vi "AOI - PCB.vi"() -> ()   [LabVIEW 2017]
doc: "Printed Circuit Board Inspection\nDetermine whether PCB components are present and in the correct location using pattern matching. Match areas of inspection to a template of valid components. Use shift-invariant matching to inspect an oriented component (diode). Use rotation-invariant matching to inspect an unoriented component (resistor)."
panel:
  out "Image":T1(plugin-control)
  out "Not found 1":bool
  out "Not found 2":bool
  out "Number of Matches 2":i32
  out "Number of Matches1":i32
  in  "Template File path 1":path=path "c:/vision/AOI/Template Diode.png"
  in  "Template File path 2":path=path "c:/vision/AOI/Template Resistor.png"
  in  "Image File path":path=path "c:/vision/AOI/SMD Diodes 01.jpg"
  out "Image Log path":path=path "c:/vision/Result.jpg"
  out "error out":errorcluster
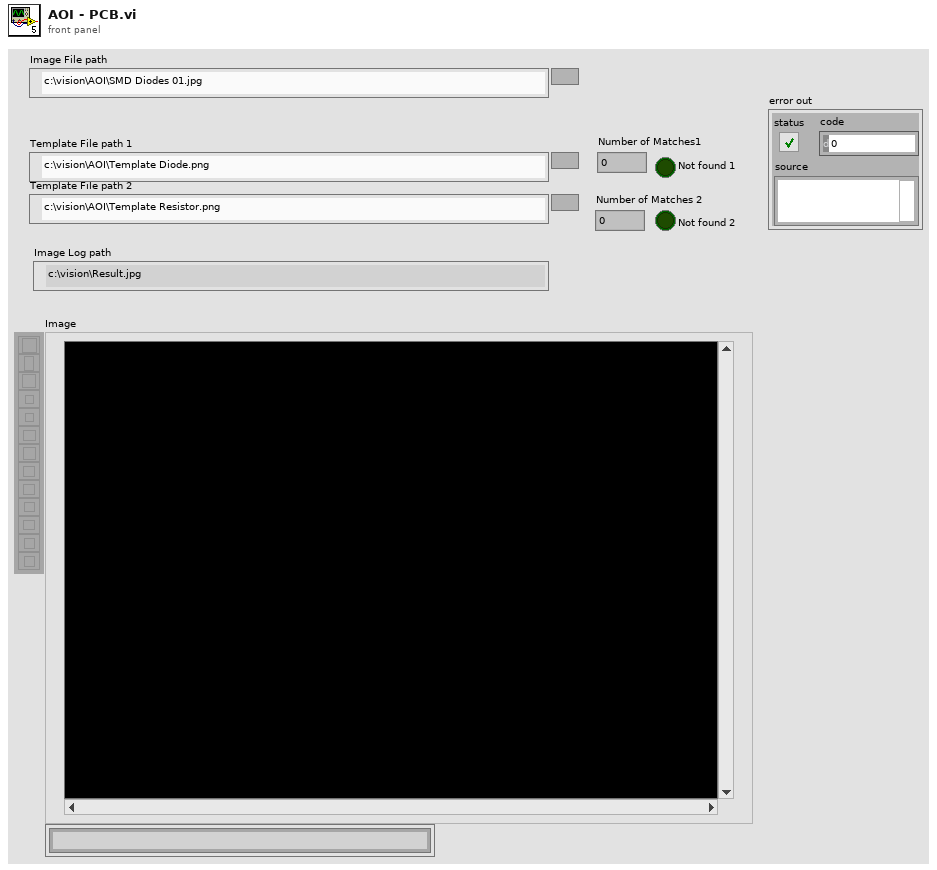
[diagram p1: front panel]
types:
  T1 = typedef "IMAQ Image.ctl" = refnum<image>
  T2 = cluster{"Global Rectangle":i32[], "Contours":cluster{"ID":enum32{"External", "Internal"}, "Type":u32, "Coordinates":i32[]}[]}
  T3 = typedef "Image Type" = u32
  T4 = cluster{"Position":cluster{"x":sgl, "y":sgl}, "Angle":sgl, "Scale":sgl, "Score":sgl, "Bounding Box":cluster{"x":sgl, "y":sgl}[]}[]
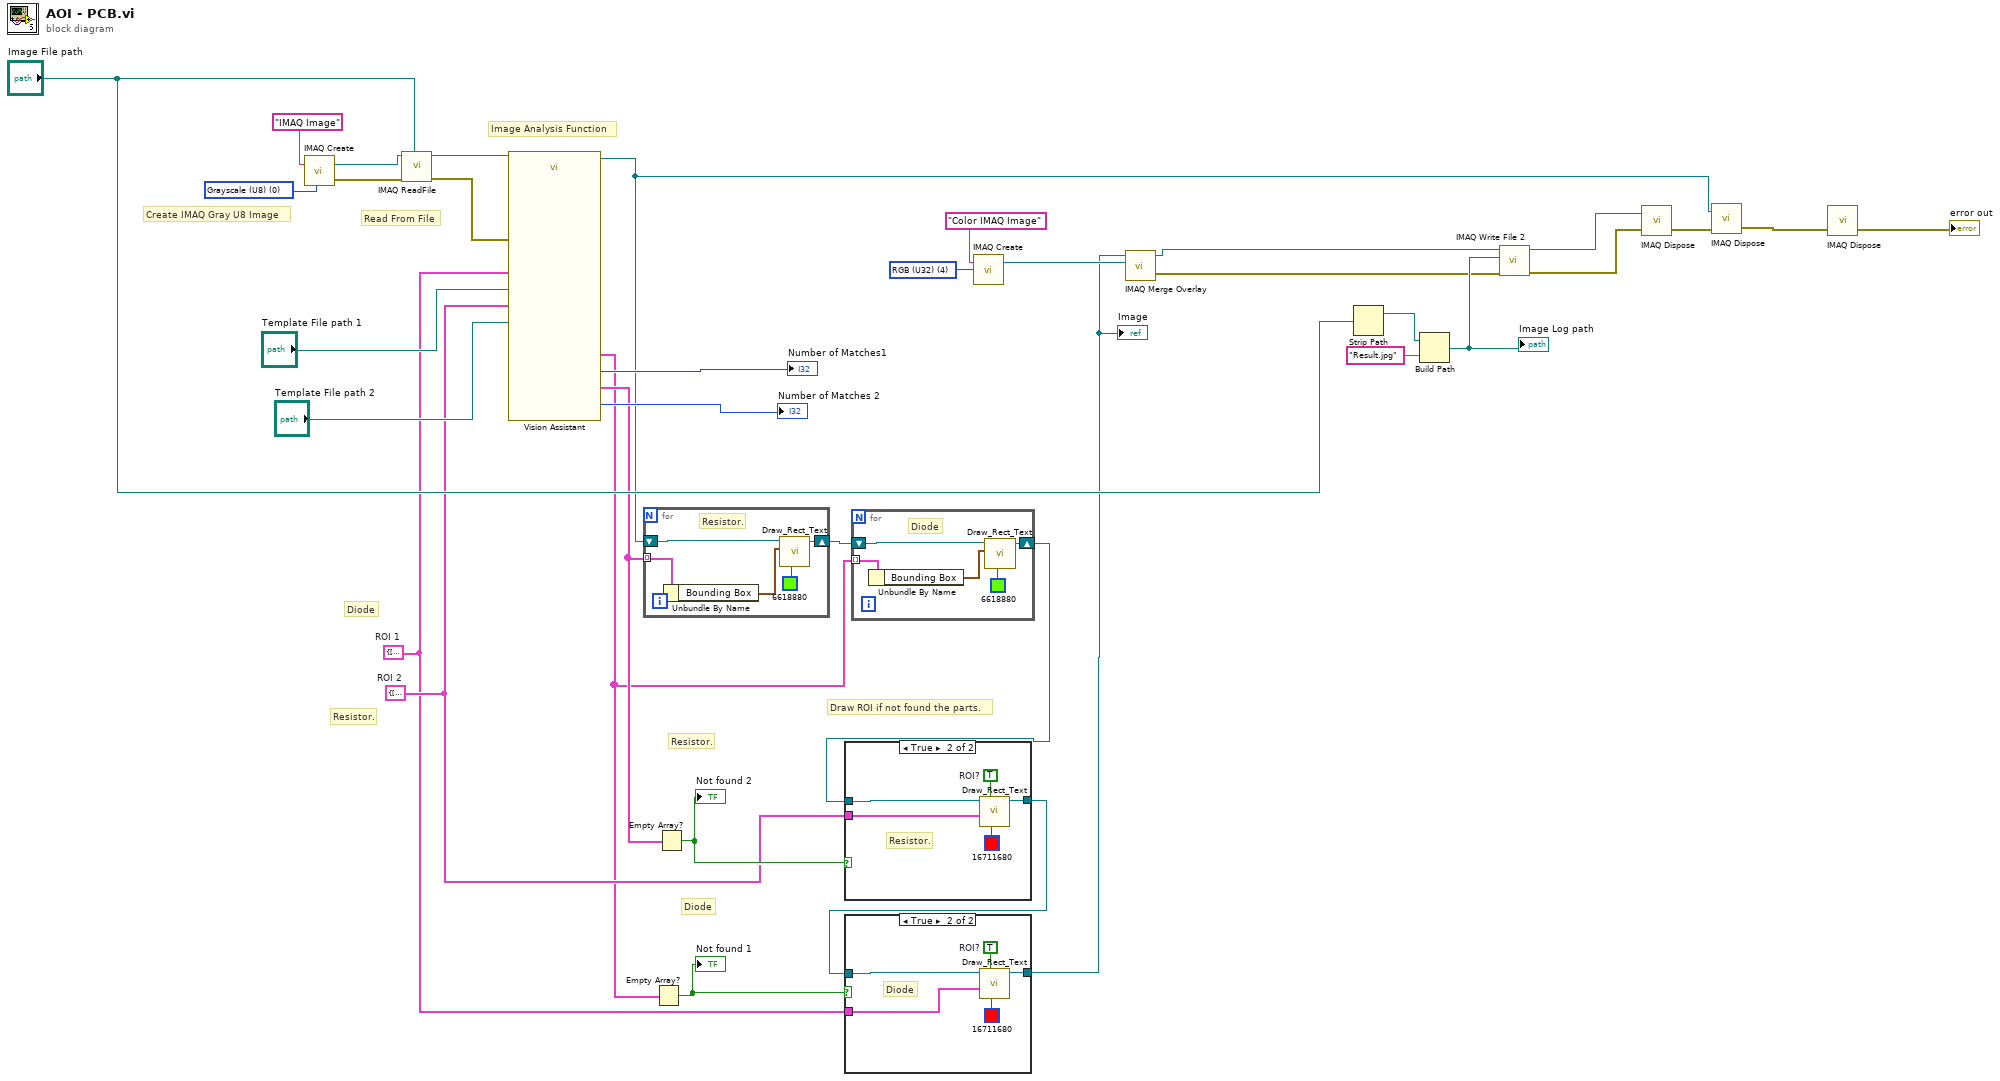
[diagram p0: block diagram]
diagram:
  w7 = T2 {"Global Rectangle"=[154, 137, 231, 181], "Contours"=[{"ID"=enum."External", "Type"=12, "Coordinates"=[154, 137, 231, 181, 0]}]}  # ROI 2
  w3 = T2 {"Global Rectangle"=[340, 217, 376, 284], "Contours"=[{"ID"=enum."External", "Type"=12, "Coordinates"=[340, 217, 376, 284, 0]}]}  # ROI 1
  w28 = T3 4 items=["Grayscale (U8)", "Grayscale (I16)", "Grayscale (SGL)", "Complex (CSG)", "RGB (U32)", "HSL (U32)", "RGB (U64)", "Grayscale (U16)"] ("Image Type")
  w32 = T3 0 items=["Grayscale (U8)", "Grayscale (I16)", "Grayscale (SGL)", "Complex (CSG)", "RGB (U32)", "HSL (U32)", "RGB (U64)", "Grayscale (U16)"] ("Image Type")
  # "Draw ROI if not found the parts."
  # "Resistor."
  # "Diode"
  # "Diode"
  # "Resistor."
  # "Image Analysis Function"
  # "Read From File"
  # "Create IMAQ Gray U8 Image"
  n1 = call "IMAQ Create"("Image Name"="IMAQ Image", "Image Type"=w32) -> ("New Image"=w34:T1, "error out"=w33:errorcluster)  [unwired: 2 in, 1 out]
  n2 = call "IMAQ ReadFile"("File Path"="Image File path", "error in (no error)"=w33, "Image"=w34) -> ("error out"=w30:errorcluster, "Image Out"=w12:T1)  [unwired: 2 in, 5 out]
  n3 = call "Vision Assistant"("Image In"=w12, "Template File Path (Pattern Matching 1)"="Template File path 1", "Template File Path (Pattern Matching 2)"="Template File path 2", "ROI Descriptor (Pattern Matching 1)"=w3, "ROI Descriptor (Pattern Matching 2)"=w7, "error in"=w30) -> ("Image Out"=w13:T1, "Matches (Pattern Matching 1)"=w6:T4, "Number of Matches (Pattern Matching 1)"=→"Number of Matches1":i32, "Matches (Pattern Matching 2)"=w10:T4, "Number of Matches (Pattern Matching 2)"=→"Number of Matches 2":i32)  [unwired: 16 in, 1 out]
  n4 = for {
    tunnel: w10 -> [w40] mode=indexing
    shift-right: [w36] -> w11
    shift-left: w13 -> [w39]
    # "Resistor."
    n5 = Unbundle By Name(w40) -> ("Bounding Box"=w38:cluster{"x":sgl, "y":sgl}[])
    n6 = call "Draw_Rect_Text.vi"("Color"=u32 6618880, "Bounding Box"=w38, "Image"=w39) -> ("Image 2"=w36:T1)  [unwired: 7 in, 1 out]
  }
  n7 = Empty Array?(array=w6) -> (empty?=w2:bool)
  "Not found 1" <- w2
  n8 = Empty Array?(array=w10) -> (empty?=w8:bool)
  "Not found 2" <- w8
  n9 = for {
    tunnel: w6 -> [w45] mode=indexing
    shift-right: [w41] -> w9
    shift-left: w11 -> [w44]
    # "Diode"
    n10 = Unbundle By Name(w45) -> ("Bounding Box"=w42:cluster{"x":sgl, "y":sgl}[])
    n11 = call "Draw_Rect_Text.vi"("Color"=u32 6618880, "Bounding Box"=w42, "Image"=w44) -> ("Image 2"=w41:T1)  [unwired: 7 in, 1 out]
  }
  n12 = case shown="True" w8 {
    tunnel: w9 -> [w46 w51]
    tunnel: w7 -> [_ w48]
    tunnel: [w46 w47] -> w5
    frame False {
    }
    frame True {
      w49 = TRUE  # ROI?
      # "Resistor."
      n13 = call "Draw_Rect_Text.vi"("Color"=u32 16711680, "ROI?"=w49, "RIO Input"=w48, "Image"=w51) -> ("Image 2"=w47:T1)  [unwired: 6 in, 1 out]
    }
  }
  n14 = case shown="True" w2 {
    tunnel: w5 -> [w52 w57]
    tunnel: [w52 w54] -> w4
    tunnel: w3 -> [_ w53]
    frame False {
    }
    frame True {
      w55 = TRUE  # ROI?
      # "Diode"
      n15 = call "Draw_Rect_Text.vi"("Color"=u32 16711680, "ROI?"=w55, "RIO Input"=w53, "Image"=w57) -> ("Image 2"=w54:T1)  [unwired: 6 in, 1 out]
    }
  }
  "Image" <- w4
  n16 = call "IMAQ Create"("Image Name"="Color IMAQ Image", "Image Type"=w28) -> ("New Image"=w27:T1)  [unwired: 2 in, 2 out]
  n17 = call "IMAQ Merge Overlay"("Image Dst"=w27, "Image Src"=w4) -> ("error out"=w14:errorcluster, "Image Dst Out"=w26:T1)  [unwired: 8 in]
  n18 = Strip Path(path="Image File path") -> (stripped path=w24:path)  [unwired: 1 out]
  n19 = Build Path(base path=w24, name or relative path="Result.jpg") -> (appended path=w22:path)
  "Image Log path" <- w22
  n20 = call-poly "IMAQ Write File 2"("error in (no error)"=w14, "File Path"=w22, "Image"=w26) -> ("error out"=w15:errorcluster, "Image Out (duplicate)"=w16:T1)  [unwired: 7 in]
  n21 = call "IMAQ Dispose"("Image"=w16, "error in (no error)"=w15) -> ("error out"=w17:errorcluster)  [unwired: 4 in]
  n22 = call "IMAQ Dispose"("Image"=w13, "error in (no error)"=w17) -> ("error out"=w1:errorcluster)  [unwired: 4 in]
  n23 = call "IMAQ Dispose"("error in (no error)"=w1) -> ("error out"=→"error out":errorcluster)  [unwired: 5 in]
